vi "Modified Sync Filter Weights.vi"(8 "error in (no error)":errorcluster, 10 "order (n)":i32, 11 "side points (m)":i32) -> (0 "error out":errorcluster, 3 "weights":dbl[](array[numeric]))   [LabVIEW 2021, in "Math.lvlib"]
uses:
  Math.lvlib
  3c26feb9-706f-47a2-9a11-bbc09564da1d.vi
  50009ead-77da-4d6c-99ce-cc0555d7abd4.vi
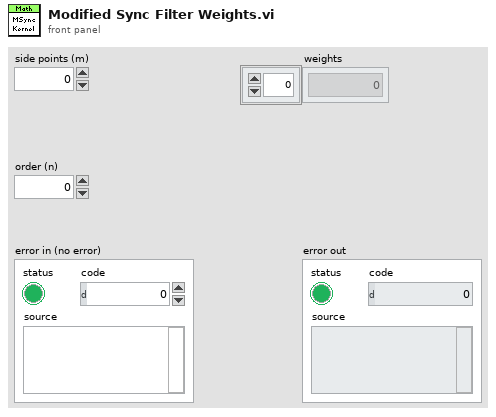
[diagram p1: front panel]
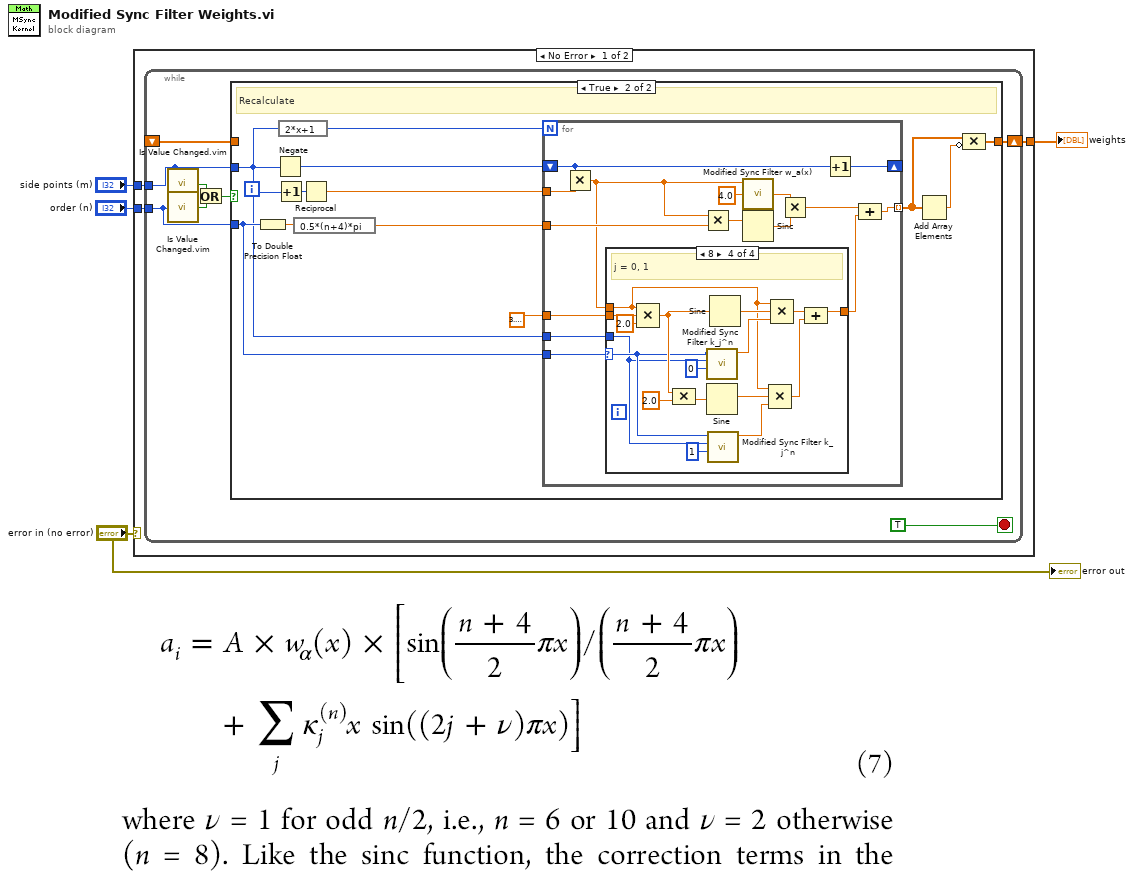
[diagram p0: block diagram]
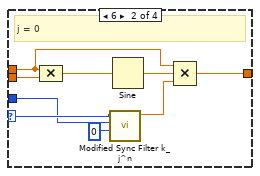
[diagram p4: hidden frame]
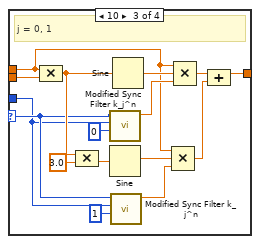
[diagram p5: hidden frame]
diagram:
  n1 = case shown="No Error" "error in (no error)" {
    tunnel: "side points (m)" -> [w7 _]
    tunnel: "order (n)" -> [w6 _]
    tunnel: [w5 _] -> w1
    frame No Error {
      n2 = while {
        tunnel: w7 -> [w10]
        tunnel: w6 -> [w9]
        shift-right: [w8] -> w5
        shift-left: _ -> [w11]
        stop <- TRUE stop-if-true
        n3 = call "Is Value Changed.vim"("value"=w10) -> ("changed or first call?"=w14:bool)
        n4 = call "Is Value Changed.vim"("value"=w9) -> ("changed or first call?"=w13:bool)
        n5 = Or(x=w14, y=w13) -> (x .or. y?=w12:bool)
        n6 = case shown="True" w12 {
          tunnel: w11 -> [w16 _]
          tunnel: [w16 w21] -> w8
          tunnel: w10 -> [_ w17]
          tunnel: w9 -> [_ w19]
          frame False {
            # "Use stored weights"
          }
          frame True {
            # "Recalculate"
            n7 = To Double Precision Float(number=w19) -> (double precision float=w23:dbl)
            n8 = Negate(x=w17) -> (-x=w28:i32)
            n9 = Increment(x=w17) -> (x+1=w26:i32)
            n10 = expression code="2*x+1"(w17) -> (w27:i32)
            n11 = expression code="0.5*(n+4)*pi"(w23) -> (w24:dbl)
            n12 = Reciprocal(x=w26) -> (1/x=w25:dbl)
            n13 = for {
              N: w27 -> [_]
              shift-right: [w43] -> _
              shift-left: w28 -> [w41]
              tunnel: w25 -> [w42]
              tunnel: w24 -> [w39]
              tunnel: [w34] -> w22 mode=indexing
              tunnel: w19 -> [w33]
              tunnel: 3.141592653589793 -> [w30]
              tunnel: w17 -> [w29]
              n14 = Multiply(x=w41, y=w42) -> (x*y=w32:dbl)
              n15 = case shown="8" w33 {
                selector: w33 -> [_ w47 w58 w75]
                tunnel: w32 -> [_ w48 w59 w76]
                tunnel: [_ w49 w54 w71] -> w31
                tunnel: w30 -> [_ w51 w68 w85]
                tunnel: w29 -> [_ w46 w57 w74]
                frame 0, Default {
                }
                frame 6 {
                  # "j = 0"
                  n16 = Compound Arithmetic op=MULTIPLY(w48, w51) -> (w52:dbl)
                  n17 = call "Modified Sync Filter k_j^n.vi"("j"=0, "m"=w46, "n"=w47) -> ("k_j^(n)"=w44:dbl)  [unwired: 8 in]
                  n18 = Sine(x=w52) -> (sin(x)=w50:dbl)
                  n19 = Compound Arithmetic op=MULTIPLY(w48, w50, w44) -> (w49:dbl)
                }
                frame 10 {
                  # "j = 0, 1"
                  n20 = Compound Arithmetic op=MULTIPLY(w59, w68) -> (w63:dbl)
                  n21 = Compound Arithmetic op=MULTIPLY(w63, 3.0 ("value")) -> (w61:dbl)
                  n22 = call "Modified Sync Filter k_j^n.vi"("j"=0, "m"=w57, "n"=w58) -> ("k_j^(n)"=w64:dbl)  [unwired: 8 in]
                  n23 = Sine(x=w61) -> (sin(x)=w60:dbl)
                  n24 = call "Modified Sync Filter k_j^n.vi"("j"=1, "m"=w57, "n"=w58) -> ("k_j^(n)"=w55:dbl)  [unwired: 8 in]
                  n25 = Sine(x=w63) -> (sin(x)=w67:dbl)
                  n26 = Compound Arithmetic op=MULTIPLY(w59, w60, w55) -> (w53:dbl)
                  n27 = Compound Arithmetic op=MULTIPLY(w59, w67, w64) -> (w66:dbl)
                  n28 = Compound Arithmetic op=ADD(w66, w53) -> (w54:dbl)
                }
                frame 8 {
                  # "j = 0, 1"
                  n29 = Compound Arithmetic op=MULTIPLY(w76, w85, 2.0 ("value")) -> (w80:dbl)
                  n30 = Compound Arithmetic op=MULTIPLY(w80, 2.0 ("value")) -> (w78:dbl)
                  n31 = call "Modified Sync Filter k_j^n.vi"("j"=0, "m"=w74, "n"=w75) -> ("k_j^(n)"=w81:dbl)  [unwired: 8 in]
                  n32 = Sine(x=w78) -> (sin(x)=w77:dbl)
                  n33 = call "Modified Sync Filter k_j^n.vi"("j"=1, "m"=w74, "n"=w75) -> ("k_j^(n)"=w72:dbl)  [unwired: 8 in]
                  n34 = Sine(x=w80) -> (sin(x)=w84:dbl)
                  n35 = Compound Arithmetic op=MULTIPLY(w76, w77, w72) -> (w70:dbl)
                  n36 = Compound Arithmetic op=MULTIPLY(w76, w84, w81) -> (w83:dbl)
                  n37 = Compound Arithmetic op=ADD(w83, w70) -> (w71:dbl)
                }
              }
              n38 = Multiply(x=w32, y=w39) -> (x*y=w38:dbl)
              n39 = call "Modified Sync Filter w_a(x).vi"("x(i)"=w32, "alpha"=4.0) -> ("w_a(x)"=w37:dbl)  [unwired: 7 in]
              n40 = Sinc(1:w38) -> (0:w36:dbl)
              n41 = Multiply(x=w37, y=w36) -> (x*y=w35:dbl)
              n42 = Increment(x=w41) -> (x+1=w43:i32)
              n43 = Compound Arithmetic op=ADD(w35, w31) -> (w34:dbl)
            }
            n44 = Add Array Elements(numeric array=w22) -> (sum=w20:dbl)
            n45 = Compound Arithmetic op=MULTIPLY(w22, invert w20) -> (w21:dbl[])
          }
        }
      }
    }
    frame Error {
    }
  }
  "weights" <- w1
  "error out" <- "error in (no error)"
